vi "omega map fit function.vi"(3 "output control":T1, 4 "data":T2, 5 "X":dbl[](array[numeric]), 6 "a":dbl[](array[numeric])) -> (0 "error out":errorcluster, 1 "f'(X,a)":dbl[][](array[numeric]), 2 "f(X,a)":dbl[](array[numeric]))   [LabVIEW 2015]
doc: "This template is the starting point for creating a model function to be passed to the Nonlinear Curve Fit.vi."
uses:
  <vilib>/gmath/NumericalOptimization/objective function data.ctl
  <vilib>/gmath/NumericalOptimization/LM_output select.ctl
  <vilib>/gmath/NI_Gmath.lvlib
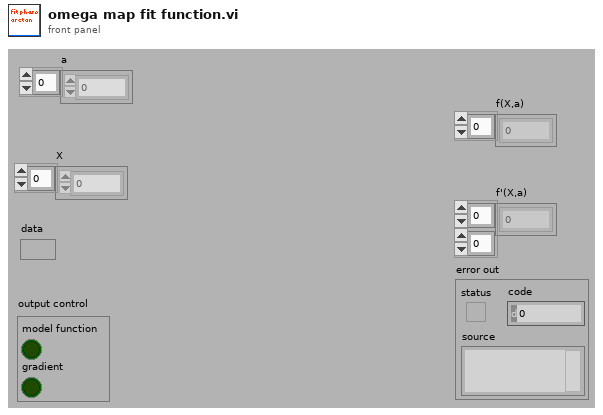
[diagram p1: front panel]
types:
  T1 = typedef "NI_Gmath.lvlib/LM_output select.ctl" = cluster{"model function":bool, "gradient":bool}
  T2 = typedef "NI_Gmath.lvlib/objective function data.ctl" = variant
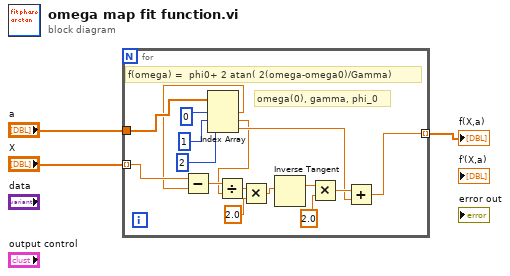
[diagram p0: block diagram]
diagram:
  n1 = for {
    tunnel: "a" -> [w18]
    tunnel: "X" -> [w14] mode=indexing
    tunnel: [w8] -> w1 mode=indexing
    # "f(omega) =  phi0+ 2 atan( 2(omega-omega0)/Gamma)"
    # "omega(0), gamma, phi_0"
    n2 = Index Array(array=w18, index #1=0 ("index"), index #2=1 ("index"), index #3=2 ("index")) -> (element #1=w13:dbl, element #2=w7:dbl, element #3=w9:dbl)
    n3 = Subtract(x=w14, y=w13) -> (x-y=w12:dbl)
    n4 = Divide(x=w12, y=w7) -> (x/y=w4:dbl)
    n5 = Multiply(x=w4, y=2.0) -> (x*y=w5:dbl)
    n6 = Inverse Tangent(1:w5) -> (0:w11:dbl)
    n7 = Multiply(x=w11, y=2.0) -> (x*y=w10:dbl)
    n8 = Add(x=w10, y=w9) -> (x+y=w8:dbl)
  }
  "f(X,a)" <- w1
